vi "Calc_R_Alpha.vi"(0 "Mode":enum16{"Initialize", "Calculate"}(ring), 2 "Config file name":path=path "C:/Users/ceslab/Documents/CES LabView/Configuration/CES_Config_test.ini", 3 "Pressure in":dbl, 4 "Temperature In":dbl, 5 "error in":errorcluster, 7 "Wavelength":dbl[](array[numeric]), 8 "State in":i32, 9 "Spectra":dbl[](array[numeric])) -> (13 "NO2 Conc (ppb)":dbl, 14 "Rs":cluster{"Wavelength":dbl[], "Array out":dbl[]}, 15 "Exts":cluster{"Wavelength":dbl[], "Array out":dbl[]}, 16 "First?":bool, 17 "Darks":cluster{"Wavelength":dbl[], "Ch1 Dark":dbl[]}, 18 "Gly Conc (ppb)":dbl, 19 "error out":errorcluster)   [LabVIEW 2025]
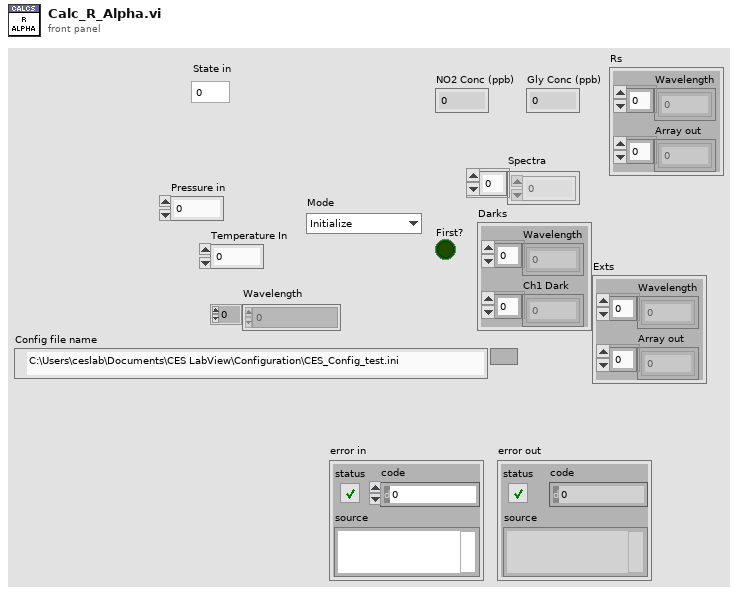
[diagram p1: front panel]
types:
  T1 = enum16{"Spectrometer", "Calculations", "BBB", "States", "Actions"}
  T2 = typedef "TypeDef_SpectrometerConfigData.ctl" = cluster{"pixels":i32, "start wavelength":dbl, "stop wavelength":dbl}
  T3 = typedef "TypeDef_CalculationConfigData.ctl" = cluster{"Cavity_length":dbl, "Pre_dark":i32, "Dark":i32, "Pre_R":i32, "R":i32, "Pre_Zero":i32, "Zero":i32, "Start_pixel":i32, "Stop_pixel":i32}
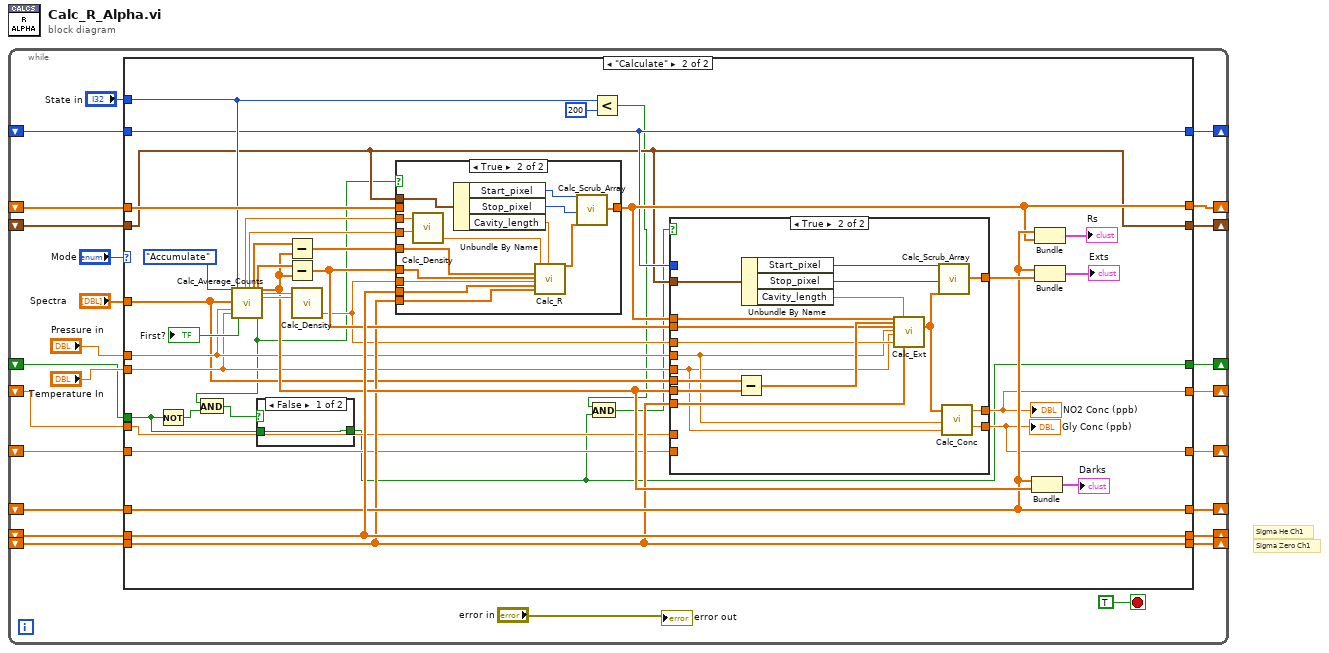
[diagram p0: block diagram]
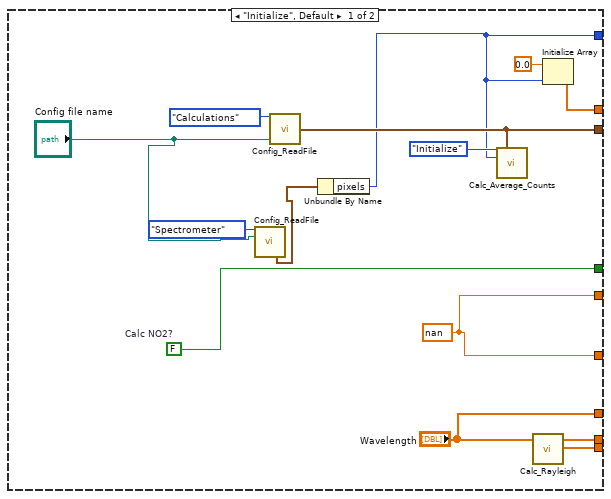
[diagram p2: hidden frame]
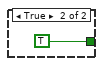
[diagram p3: hidden frame]
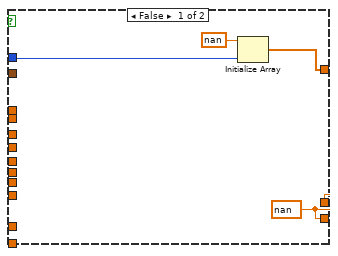
[diagram p4: hidden frame]
diagram:
  # "Sigma Zero Ch1"
  # "Sigma He Ch1"
  n1 = while {
    shift-right: [w23] -> _
    shift-left: _ -> [w21]
    shift-right: [w22] -> _
    shift-left: _ -> [w20]
    shift-right: [w18] -> _
    shift-left: _ -> [w17]
    shift-right: [w15] -> _
    shift-left: _ -> [w14]
    shift-right: [w11] -> _
    shift-left: _ -> [w10]
    shift-right: [w8] -> _
    shift-left: _ -> [w7]
    shift-right: [w6] -> _
    shift-left: _ -> [w5]
    shift-right: [w4] -> _
    shift-left: _ -> [w3]
    shift-right: [w2] -> _
    shift-left: _ -> [w1]
    stop <- TRUE stop-if-true
    n2 = case shown="\"Calculate\"" "Mode" {
      tunnel: [w39 w75] -> w23
      tunnel: [w38 w59] -> w22
      tunnel: w21 -> [_ w75]
      tunnel: w20 -> [_ w59]
      tunnel: "Spectra" -> [_ w55]
      tunnel: "Pressure in" -> [_ w57]
      tunnel: "Temperature In" -> [_ w56]
      tunnel: [w35 w61] -> w18
      tunnel: w17 -> [_ w69]
      tunnel: "State in" -> [_ w64]
      tunnel: ["Wavelength" w62] -> w15
      tunnel: w14 -> [_ w62]
      tunnel: [w31 w52] -> w11
      tunnel: w10 -> [_ w52]
      tunnel: [w32 w51] -> w8
      tunnel: w7 -> [_ w51]
      tunnel: [w27 w50] -> w6
      tunnel: w5 -> [_ w49]
      tunnel: [w27 w48] -> w4
      tunnel: w3 -> [_ w47]
      tunnel: [w26 w42] -> w2
      tunnel: w1 -> [_ w40]
      frame "Initialize", Default {
        w26 = FALSE  # Calc NO2?
        w27 = nan
        n3 = call "Config_ReadFile.vi"("Section"=T1."Spectrometer", "Config file name"="Config file name") -> ("Spectrometer config data"=w28:T2)  [unwired: 7 in, 6 out]
        n4 = call "Config_ReadFile.vi"("Section"=T1."Calculations", "Config file name"="Config file name") -> ("Calculation config data"=w32:T3)  [unwired: 7 in, 6 out]
        n5 = Unbundle By Name(w28) -> ("pixels"=w31:i32)
        n6 = call "Calc_Average_Counts.vi"("Mode"=enum16{"Initialize", "Accumulate"}."Initialize", "NumPixels"=w31, "Calculation config data"=w32) -> ()  [unwired: 15 in, 10 out]
        n7 = call "Calc_Rayleigh.vi"("Wavelength"="Wavelength") -> ("Rayleigh He"=w39:dbl[], "Rayleigh Ambient"=w38:dbl[])  [unwired: 25 in]
        n8 = Initialize Array(0.0 ("element"), w31) -> (w35:dbl[])
      }
      frame "Calculate" {
        n9 = Not(x=w40) -> (.not. x?=w45:bool)
        n10 = call "Calc_Average_Counts.vi"("Mode"=enum16{"Initialize", "Accumulate"}."Accumulate", "Spectra"=w55, "Pressure in"=w57, "Temperature in"=w56, "State in"=w64) -> ("First?"=→"First?":bool, "Pressure during R"=w77:dbl, "Temperature during R"=w76:dbl, "R counts"=w74:dbl[], "Zero counts"=w73:dbl[], "Calc R?"=w46:bool, "Ch1 Dark"=w63:dbl[], "Pressure during Zero"=w72:dbl, "Temperature during Zero"=w71:dbl)  [unwired: 13 in, 1 out]
        n11 = And(x=w46, y=w45) -> (x .and. y?=w44:bool)
        n12 = case shown="False" w44 {
          tunnel: [w79 TRUE] -> w42
          tunnel: w40 -> [w79 _]
          frame False {
          }
          frame True {
          }
        }
        n13 = Subtract(x=w74, y=w63) -> (x-y=w70:dbl[])
        n14 = Subtract(x=w73, y=w63) -> (x-y=w68:dbl[])
        n15 = call "Calc_Density.vi"("Pres (hPa)"=w72, "T (C)"=w71) -> ("Density (cm^-3)"=w58:dbl)  [unwired: 25 in]
        n16 = case shown="True" w46 {
          tunnel: w77 -> [_ w116]
          tunnel: w76 -> [_ w115]
          tunnel: w75 -> [_ w114]
          tunnel: w59 -> [_ w113]
          tunnel: w70 -> [_ w112]
          tunnel: w68 -> [_ w111]
          tunnel: w58 -> [_ w109]
          tunnel: w69 -> [w102 _]
          tunnel: [w102 w106] -> w61
          tunnel: w51 -> [_ w108]
          frame False {
          }
          frame True {
            n17 = call "Calc_Density.vi"("Pres (hPa)"=w116, "T (C)"=w115) -> ("Density (cm^-3)"=w110:dbl)  [unwired: 25 in]
            n18 = Unbundle By Name(w108) -> ("Start_pixel"=w105:i32, "Stop_pixel"=w104:i32, "Cavity_length"=w103:dbl)
            n19 = call "Calc_R.vi"("He_spectrum"=w112, "Zero_spectrum"=w111, "Density zero"=w109, "Rayleigh R"=w114, "Rayleigh zero"=w113, "Density R"=w110, "Length_cm"=w103) -> ("Reflectivity"=w107:dbl[])  [unwired: 20 in]
            n20 = call "Calc_Scrub_Array.vi"("Start"=w105, "Stop"=w104, "Array in"=w107) -> ("Array out"=w106:dbl[])  [unwired: 24 in]
          }
        }
        n21 = Less?(x=w64, y=200) -> (x < y?=w43:bool)
        n22 = And(x=w43, y=w42) -> (x .and. y?=w41:bool)
        n23 = case shown="True" w41 {
          tunnel: w61 -> [_ w93]
          tunnel: w63 -> [_ w101]
          tunnel: w55 -> [_ w100]
          tunnel: w68 -> [_ w94]
          tunnel: w51 -> [_ w99]
          tunnel: [w83 w96] -> w66
          tunnel: w59 -> [_ w92]
          tunnel: w58 -> [_ w91]
          tunnel: w57 -> [_ w88]
          tunnel: w56 -> [_ w86]
          tunnel: [w82 w90] -> w50
          tunnel: [w82 w89] -> w48
          tunnel: w52 -> [w81 _]
          tunnel: w49 -> [_ _]
          tunnel: w47 -> [_ _]
          frame False {
            w82 = nan ("NO2 Conc (ppb)")
            n24 = Initialize Array(nan ("element"), w81) -> (w83:dbl[])
          }
          frame True {
            n25 = Subtract(x=w100, y=w101) -> (x-y=w95:dbl[])
            n26 = Unbundle By Name(w99) -> ("Start_pixel"=w98:i32, "Stop_pixel"=w97:i32, "Cavity_length"=w85:dbl)
            n27 = call "Calc_Ext.vi"("Reflectivity"=w93, "Ambient"=w95, "I_zero"=w94, "Pressure"=w88, "Temperature"=w86, "Density zero"=w91, "Length_cm"=w85, "Rayleigh zero"=w92) -> ("Ext"=w87:dbl[])  [unwired: 19 in]
            n28 = call "Calc_Scrub_Array.vi"("Start"=w98, "Stop"=w97, "Array in"=w87) -> ("Array out"=w96:dbl[])  [unwired: 24 in]
            n29 = call "Calc_Conc.vi"("Extinction (cm-1)"=w87, "Pressure"=w88, "Temperature"=w86) -> ("NO2 Conc (ppb)"=w90:dbl, "Gly Conc (ppb)"=w89:dbl)  [unwired: 23 in]
          }
        }
        "NO2 Conc (ppb)" <- w50
        "Gly Conc (ppb)" <- w48
        n30 = Bundle("Wavelength"=w62, "Ch1 Dark"=w63) -> (→"Darks":cluster{"Wavelength":dbl[], "Ch1 Dark":dbl[]})  [unwired: 1 in]
        n31 = Bundle("Wavelength"=w62, "Array out"=w61) -> (→"Rs":cluster{"Wavelength":dbl[], "Array out":dbl[]})  [unwired: 1 in]
        n32 = Bundle("Wavelength"=w62, "Array out"=w66) -> (→"Exts":cluster{"Wavelength":dbl[], "Array out":dbl[]})  [unwired: 1 in]
      }
    }
    "error out" <- "error in"
  }
